vi "dsf show error dialog property name.vi"() -> (3 "show error property name":string)   [LabVIEW 2020, in "DSF Shared.lvlib"]
uses:
  Shared/DSF Shared.lvlib
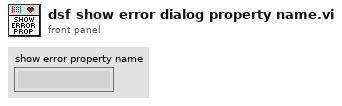
[diagram p1: front panel]
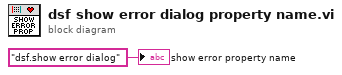
[diagram p0: block diagram]
diagram:
  "show error property name" <- "dsf.show error dialog" ("Property Name")
